vi "ExtendedKalmanFilter_SetP.vi"(10 "P":T1, 11 "in ExtendedKalmanFiilter":T2) -> (0 "Size Coerced":bool, 3 "out ExtendedKalmanFiilter":T2)   [LabVIEW 2019, in "Trajectory_Library.lvlib"]
doc: "Creates a new LINEAR SYSTEM data cluster with the specified values. \n\n\nInputs: \n - XXX -- XXX.\n\nOutputs:\n - XXX -- XXX."
uses:
  Trajectory_Library.lvlib
  EXTENDED_KALMAN_FILTER.ctl
  <vilib>/Analysis/Matrix/Datatypes/RealMatrix.ctl
  MatBuilder_Create.vi
  <vilib>/Analysis/Matrix/NI_Matrix.lvlib
panel:
  # "State Estimate <Statess,1>"
  # "<States, States>"
  # "<States, States>"
  # "<Statess,  States>"
  # "<Outputs, Outputs>"
  # "State Estimate <Statess,1>"
  # "<States, States>"
  # "<States, States>"
  # "<Statess,  States>"
  # "<Outputs, Outputs>"
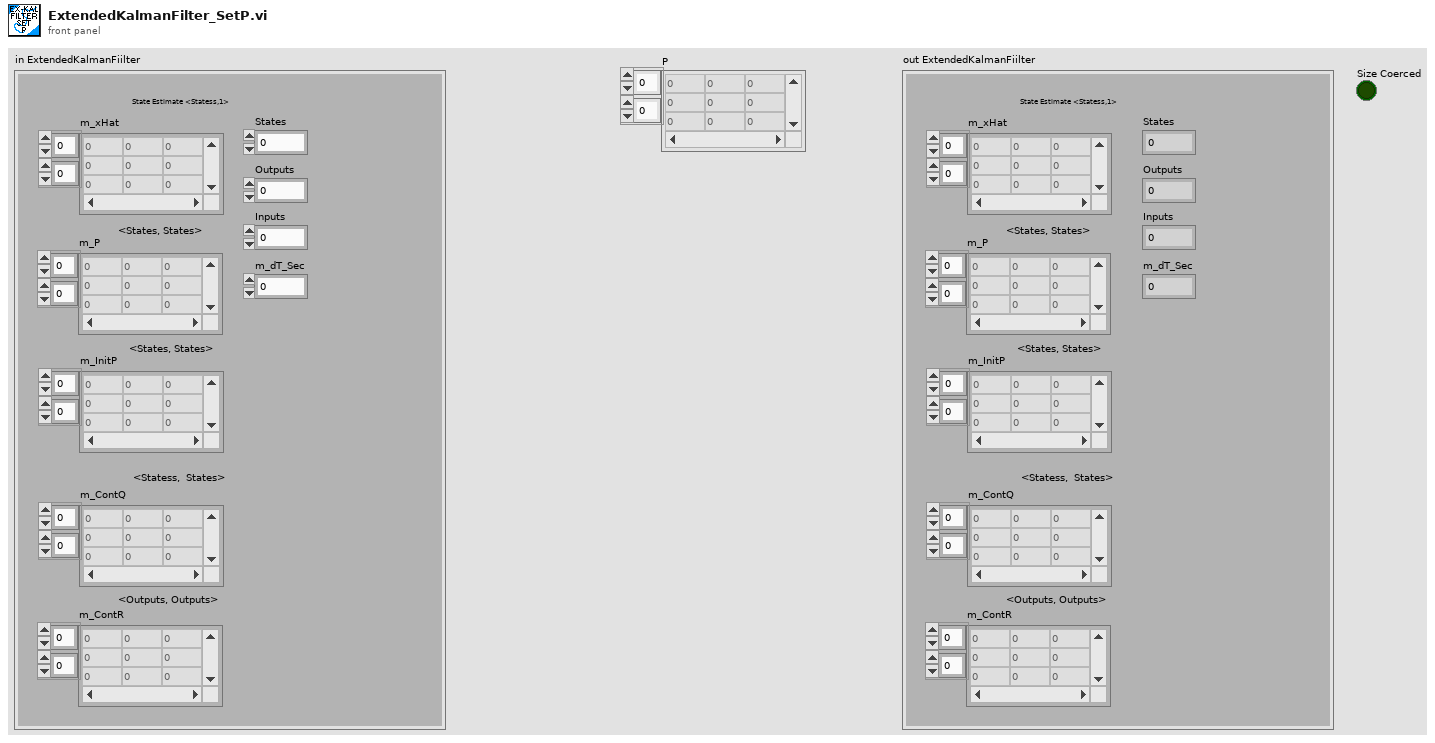
[diagram p1: front panel]
types:
  T1 = typedef "NI_Matrix.lvlib/RealMatrix.ctl" = dbl[][]
  T2 = typedef "Trajectory_Library.lvlib/EXTENDED_KALMAN_FILTER.ctl" = cluster{"m_P":T1, "m_xHat":T1, "States":i32, "Outputs":i32, "m_ContR":T1, "m_ContQ":T1, "m_dT_Sec":dbl, "Inputs":i32, "m_InitP":T1}
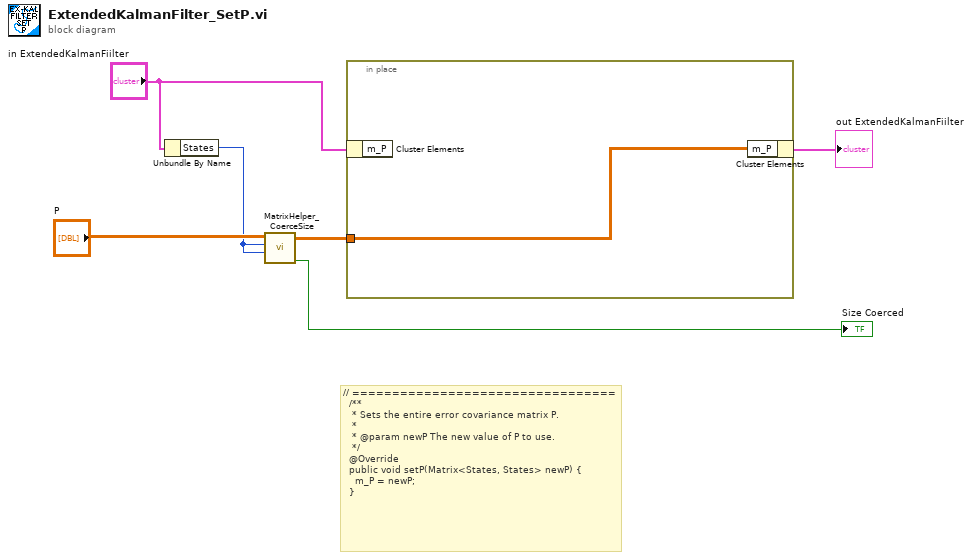
[diagram p0: block diagram]
diagram:
  # "// =================================\n  /**\n   * Sets the entire error covariance matrix P.\n   *\n   * @param newP The new value of P to use.\n   */\n  @Override\n  public void setP(Matrix<States, States> newP) {\n    m_P = newP;\n  }"
  n1 = Unbundle By Name("in ExtendedKalmanFiilter") -> ("States"=w3:i32)
  n2 = call "MatrixHelper_CoerceSize.vi"("Columns"=w3, "Rows"=w3, "input matrix"="P") -> ("Coerced"=→"Size Coerced":bool, "output matrix"=w5:T1)  [unwired: 7 in]
  n3 = in-place {
    in-place-border: w5 -> [w7]
    n4 = in-place-cluster #1("in ExtendedKalmanFiilter") -> ()  [unwired: 1 out]
    n5 = in-place-cluster #1("m_P"=w7) -> (→"out ExtendedKalmanFiilter":T2)
  }
